vi "FindBuildPath.vi"(8 "error in":errorcluster, 10 "Build Spec Name":string, 11 "Project Name":string="vicompare.lvproj") -> (0 "error out":errorcluster, 2 "Destination Path":path)   [LabVIEW 2016]
doc: "The purpose of this VI is to find the build path for a designed project and build specification. The build path is typically stored in a build specification TAG Bld_localDestDir, but it only provides an absolute path if the destination folder is above the saved project folder level. If it is adjacent or below the TAG will only give a relative path and the actual absolute path needs to be found."
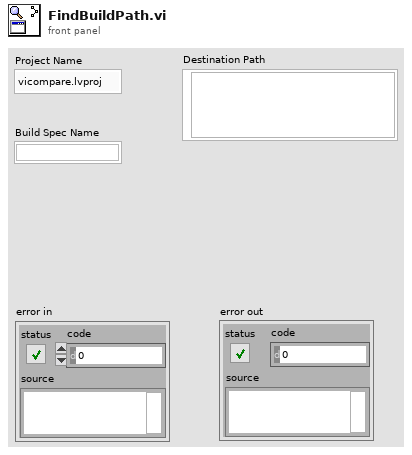
[diagram p1: front panel]
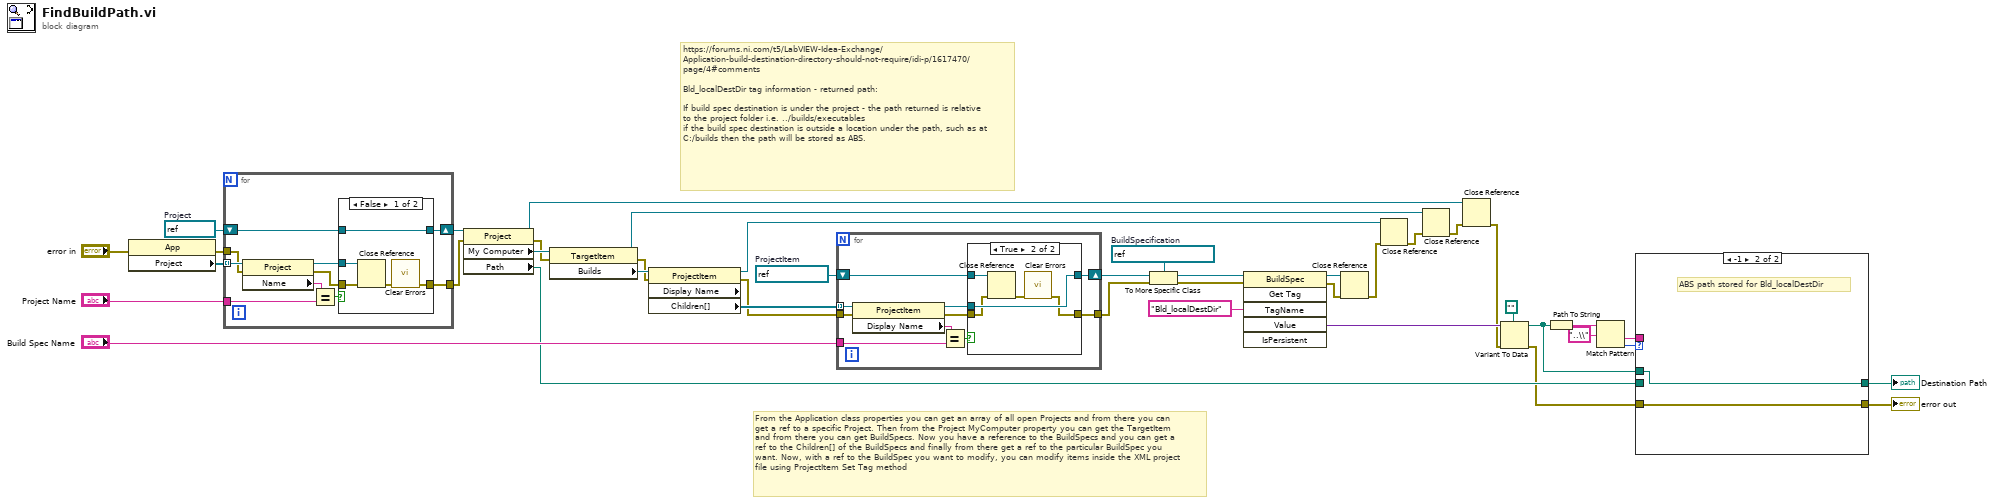
[diagram p0: block diagram]
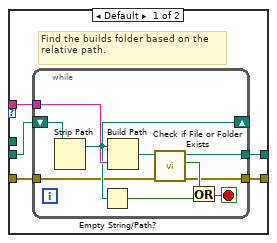
[diagram p2: hidden frame]
diagram:
  w31 = refnum<vi> refnum  # Project
  w32 = refnum<vi> refnum  # BuildSpecification
  w37 = refnum<vi> refnum  # ProjectItem
  # "https://forums.ni.com/t5/LabVIEW-Idea-Exchange/Application-build-destination-directory-should-not-require/idi-p/1617470/page/4#comments\n\nBld_localDestDir tag information - returned path:\n\nIf build spec destination is under the project - the path returned is relative to the project folder i.e. ../builds/executables\nif the build spec destination is outside a location under the path, such as at C:/builds then the path will be stored as ABS."
  # "From the Application class properties you can get an array of all open Projects and from there you can get a ref to a specific Project. Then from the Project MyComputer property you can get the TargetItem and from there you can get BuildSpecs. Now you have a reference to the BuildSpecs and you can get a ref to the Children[] of the BuildSpecs and finally from there get a ref to the particular BuildSpec you want. Now, with a ref to the BuildSpec you want to modify, you can modify items inside the XML project file using ProjectItem Set Tag method"
  n1 = property class="App"(error in="error in") -> (error out=w14:errorcluster, "Project"=w29:refnum<vi>[])  [unwired: 1 in, 1 out]
  n2 = for {
    tunnel: w29 -> [w51] mode=indexing
    tunnel: "Project Name" -> [w47]
    shift-right: [w45] -> w28
    shift-left: w31 -> [w44]
    tunnel: w14 -> [w43]
    tunnel: [w42] -> w13
    n3 = property class="Project"(reference=w51, error in=w43) -> (reference out=w49:refnum<vi>, error out=w50:errorcluster, "Name"=w46:string)
    n4 = Equal?(x=w46, y=w47) -> (x = y?=w48:bool)
    n5 = case shown="False" w48 {
      tunnel: w50 -> [w56 w57]
      tunnel: w49 -> [w55 w58]
      tunnel: [w54 w58] -> w45
      tunnel: w44 -> [w54 _]
      tunnel: [w52 w57] -> w42
      frame False {
        n6 = Close Reference(reference=w55, error in (no error)=w56) -> (error out=w53:errorcluster)
        n7 = call <vilib>:"Clear Errors.vi"("error in (no error)"=w53) -> ("error out"=w52:errorcluster)  [unwired: 5 in, 1 out]
      }
      frame True {
      }
    }
  }
  n8 = property class="Project"(reference=w28, error in=w13) -> (reference out=w21:refnum<vi>, error out=w36:errorcluster, "My Computer"=w41:refnum<vi>, "Path"=w17:path)
  n9 = property class="TargetItem"(reference=w41, error in=w36) -> (reference out=w27:refnum<vi>, error out=w35:errorcluster, "Builds"=w40:refnum<vi>)
  n10 = property class="ProjectItem" props=["Display Name", "Children[]"](reference=w40, error in=w35) -> (reference out=w8:refnum<vi>, error out=w34:errorcluster, "Children[]"=w39:refnum<vi>[])  [unwired: 1 out]
  n11 = for {
    tunnel: w39 -> [w68] mode=indexing
    tunnel: "Build Spec Name" -> [w67]
    shift-right: [w62] -> w33
    shift-left: w37 -> [w64]
    tunnel: w34 -> [w61]
    tunnel: [w60] -> w23
    n12 = property class="ProjectItem"(reference=w68, error in=w61) -> (reference out=w63:refnum<vi>, error out=w59:errorcluster, "Display Name"=w66:string)
    n13 = Equal?(x=w66, y=w67) -> (x = y?=w65:bool)
    n14 = case shown="True" w65 {
      tunnel: w64 -> [w70 w75]
      tunnel: w63 -> [_ w74]
      tunnel: [w70 w74] -> w62
      tunnel: [w69 w71] -> w60
      tunnel: w59 -> [w69 w72]
      frame False {
      }
      frame True {
        n15 = Close Reference(reference=w75, error in (no error)=w72) -> (error out=w73:errorcluster)
        n16 = call <vilib>:"Clear Errors.vi"("error in (no error)"=w73) -> ("error out"=w71:errorcluster)  [unwired: 5 in, 1 out]
      }
    }
  }
  n17 = To More Specific Class(target class=w32, reference=w33, error in=w23) -> (specific class reference=w10:refnum<vi>, error out=w9:errorcluster)
  n18 = invoke class="BuildSpec" method="Get Tag"(reference=w10, error in=w9, "TagName"="Bld_localDestDir") -> (reference out=w12:refnum<vi>, error out=w11:errorcluster, "Value"=w25:variant)  [unwired: 3 in, 3 out]
  n19 = Close Reference(reference=w12, error in (no error)=w11) -> (error out=w7:errorcluster)
  n20 = Close Reference(reference=w8, error in (no error)=w7) -> (error out=w6:errorcluster)
  n21 = Close Reference(reference=w27, error in (no error)=w6) -> (error out=w22:errorcluster)
  n22 = Close Reference(reference=w21, error in (no error)=w22) -> (error out=w5:errorcluster)
  n23 = Variant To Data(error in=w5, type=path "", Variant=w25) -> (data=w3:path, error out=w4:errorcluster)
  n24 = Path To String(path=w3) -> (string=w18:string)
  n25 = Match Pattern(string=w18, regular expression="..\\") -> (after substring=w19:string, offset past match=w16:i32)  [unwired: 1 in, 2 out]
  n26 = case shown="-1" w16 {
    tunnel: w19 -> [w80 _]
    tunnel: w17 -> [w79 _]
    tunnel: [w78 w91] -> w15
    tunnel: w4 -> [w77 w92]
    tunnel: [w76 w92] -> w2
    tunnel: w3 -> [_ w91]
    frame Default {
      # "Find the builds folder based on the relative path."
      n27 = while {
        tunnel: w80 -> [w89]
        shift-right: [w85] -> _
        shift-left: w79 -> [w90]
        tunnel: [w86] -> w78
        tunnel: w77 -> [w82]
        tunnel: [w81] -> w76
        stop <- w84 stop-if-true
        n28 = Strip Path(path=w90) -> (stripped path=w85:path)  [unwired: 1 out]
        n29 = Empty String/Path?(string/path=w85) -> (empty?=w83:bool)
        n30 = Build Path(base path=w85, name or relative path=w89) -> (appended path=w87:path)
        n31 = call <vilib>:"Check if File or Folder Exists.vi"("error in (no error)"=w82, "path"=w87) -> ("error out"=w81:errorcluster, "file or folder exists?"=w88:bool, "dup path"=w86:path)  [unwired: 7 in]
        n32 = Or(x=w88, y=w83) -> (x .or. y?=w84:bool)
      }
    }
    frame -1 {
      # "ABS path stored for Bld_localDestDir"
    }
  }
  "Destination Path" <- w15
  "error out" <- w2
